vi "Panel Washer Details.vi"(0 "Dryer In":T3 {"Cycle Count" format="%05d"}, 1 "FileName":path caption="Sample Datafilename") -> (4 "Dryer Details Out":T1, 6 "New Filenames":bool)   [LabVIEW 2009]
uses:
  Washer.ctl
  Dryer Wilt/Dryer Details.ctl
  Dryer Wilt/Globals Wilt.vi
panel:
  in  "Return":bool
  out "Array":string[][](array[string])
  out "all rows":string[][](array[string])
  in  "Read Sample Record(t, CC, Tc, ASCII, Status )":string[][](array[string])
  out "L1":dbl[](array[numeric])
  out "Time":dbl[](array[numeric])
  out "Cycle Count":dbl[](array[numeric])
  out "L2":dbl[](array[numeric])
  out "Trmb":dbl[](array[numeric])
  out "Voltage":dbl[](array[numeric])
  in  "Tab Control":T2(tab)
  out "Dryer Details":T1
  out "Display Cycle Count":i32
  out "Station Number":string
  out "Status Color":u32(colorbox)
  out "Bad Com Count":i32
  out "Com Port":u8
  out "Boolean":bool
  out "Sample Plot":cluster{dbl[], dbl[]}[](graph)
  out "Current Cycle Count":dbl
  out "I(L1),I(L2),Trmb,V.V2":dbl[][](array[numeric])
  out "Cycle Count 2":dbl[](array[numeric])
  out "Completion time":dbl[](array[numeric])
  out "L1max":dbl[](array[numeric])
  out "L2max":dbl[](array[numeric])
  out "History Plot":cluster{dbl[], dbl[]}[](graph)
  out "Tmax":dbl[](array[numeric])
  out "Serial Com Array":cluster{dbl, string}[](array[cluster]) {"?" format="%<%H:%M:%S>t"}
  out "Voltage 2":dbl[](array[numeric])
  in  "Update":bool
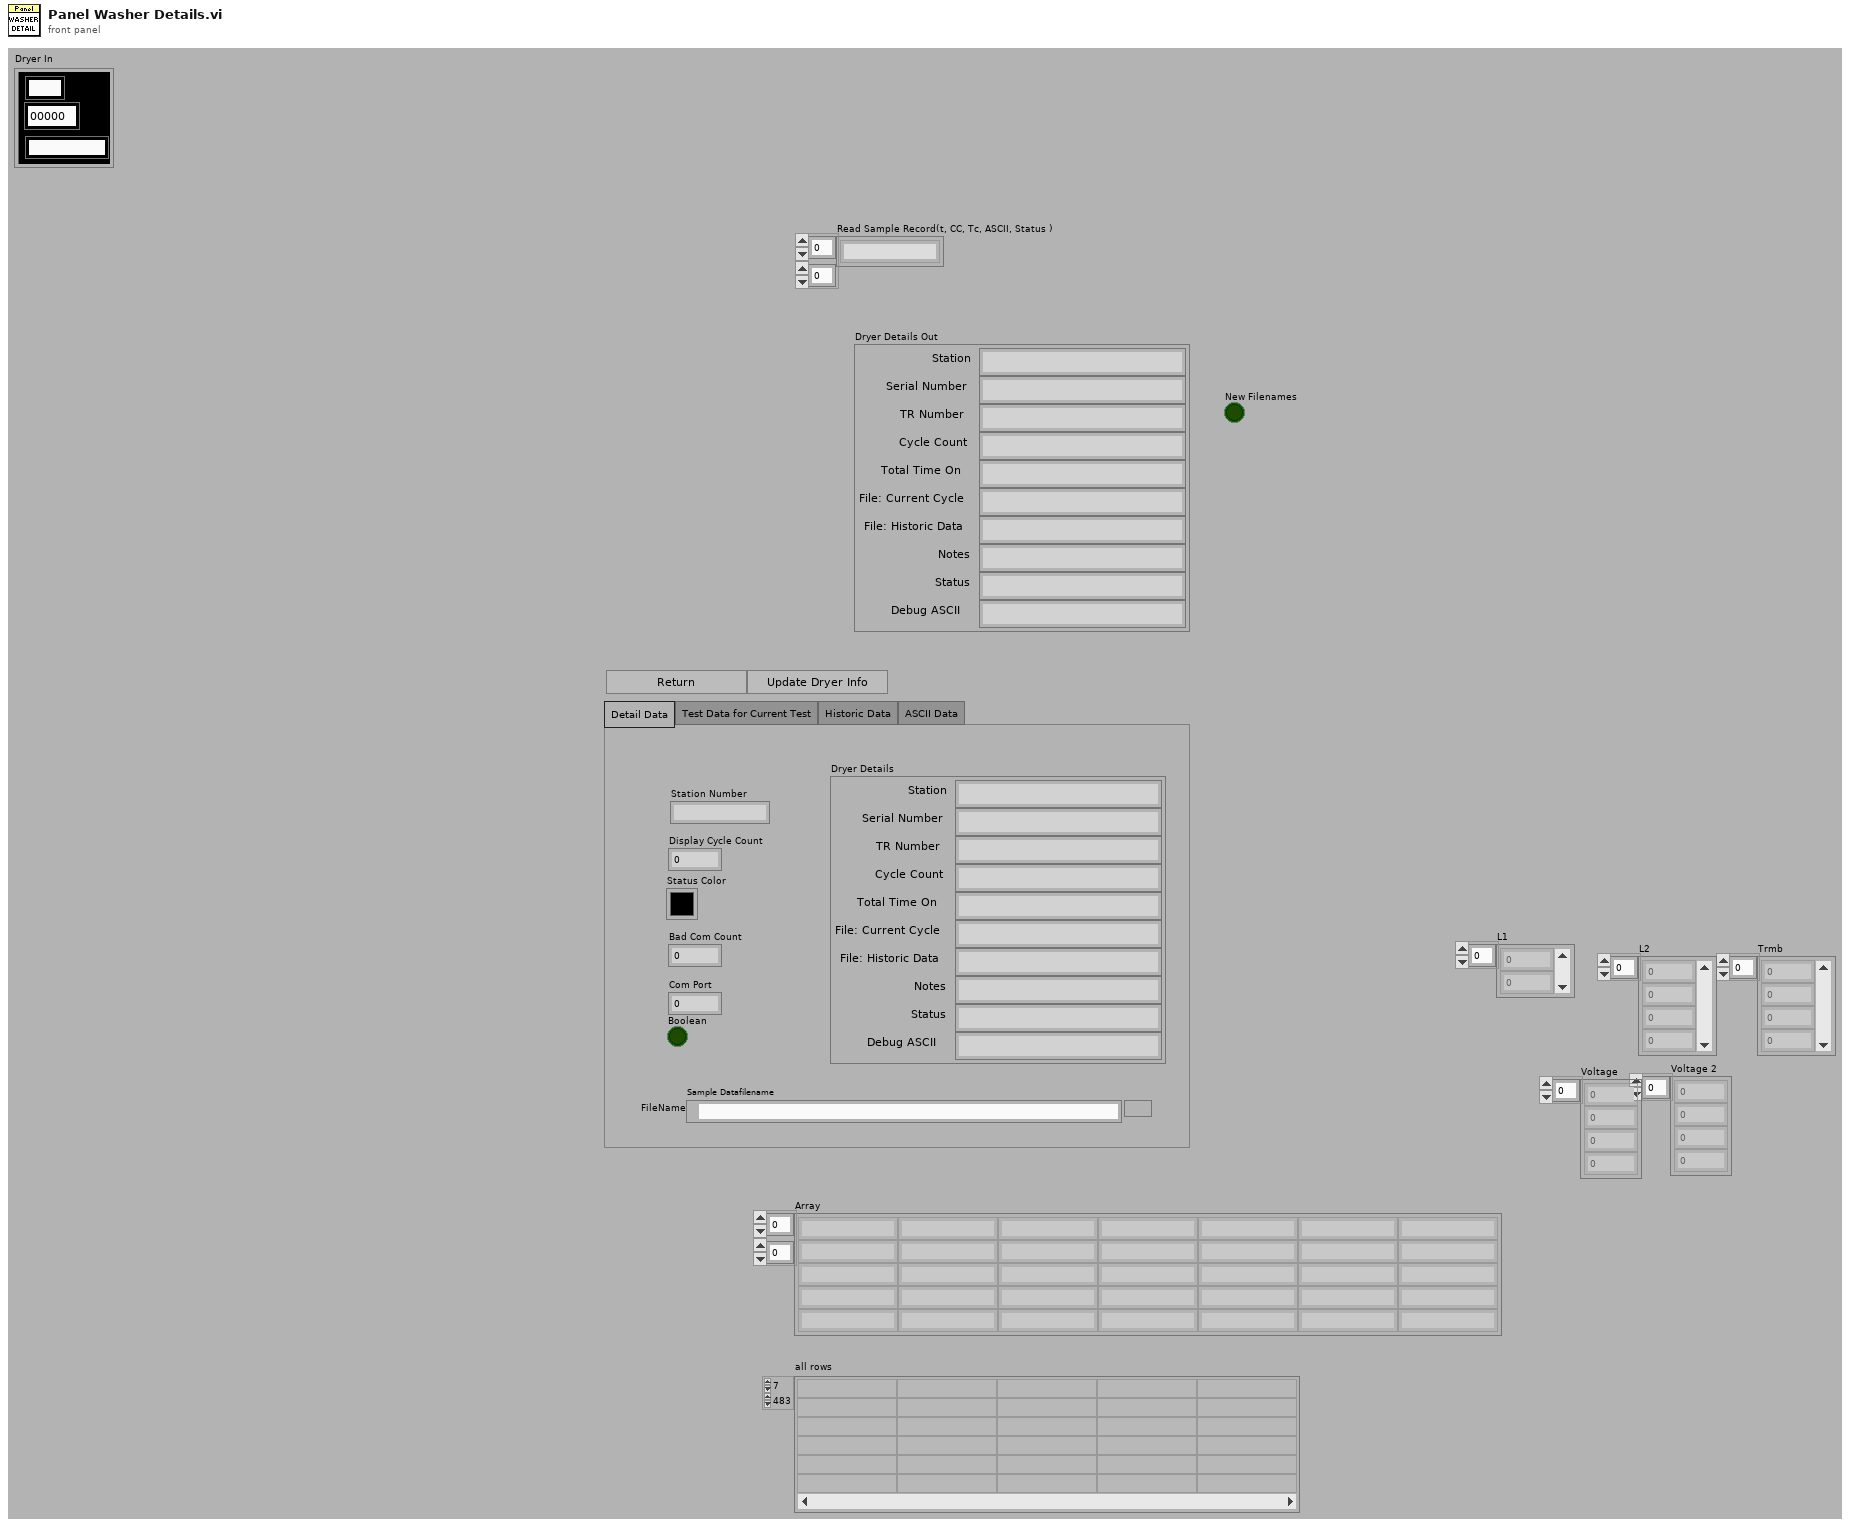
[diagram p1: front panel]
types:
  T1 = typedef "Dryer Details.ctl" = cluster{"Station":string, "Cycle Count":string, "Status":string, "Debug ASCII":string, "Notes":string, "File: Current Cycle":string, "Serial Number":string, "Total Time On":string, "TR Number":string, "File: Historic Data":string}
  T2 = enum32{"Detail Data", "Test Data for Current Test", "Historic Data", "ASCII Data"}
  T3 = typedef "Washer.ctl" = cluster{"Serial Number":string, "Cycle Count":i32, "Station Number":string, "Dryer Details":T1, "Sample Record(t, CC, ASCII, Status ) ":string[], "Hist Record(Cycle Count, t-comp) ":string[][], "Status Color":u32, "Com Port":u8, "Bad Com Count":i32, "Boolean":bool}
  T4 = enum16{"Read 2D Array", "Write 2D Array", "Write/Append 1D Array"}
  T5 = cluster{"FileName":path, "New File Info":bool, "Dryer In":T3, "Read Sample Record(t, CC, Tc, ASCII, Status )":string[][]}
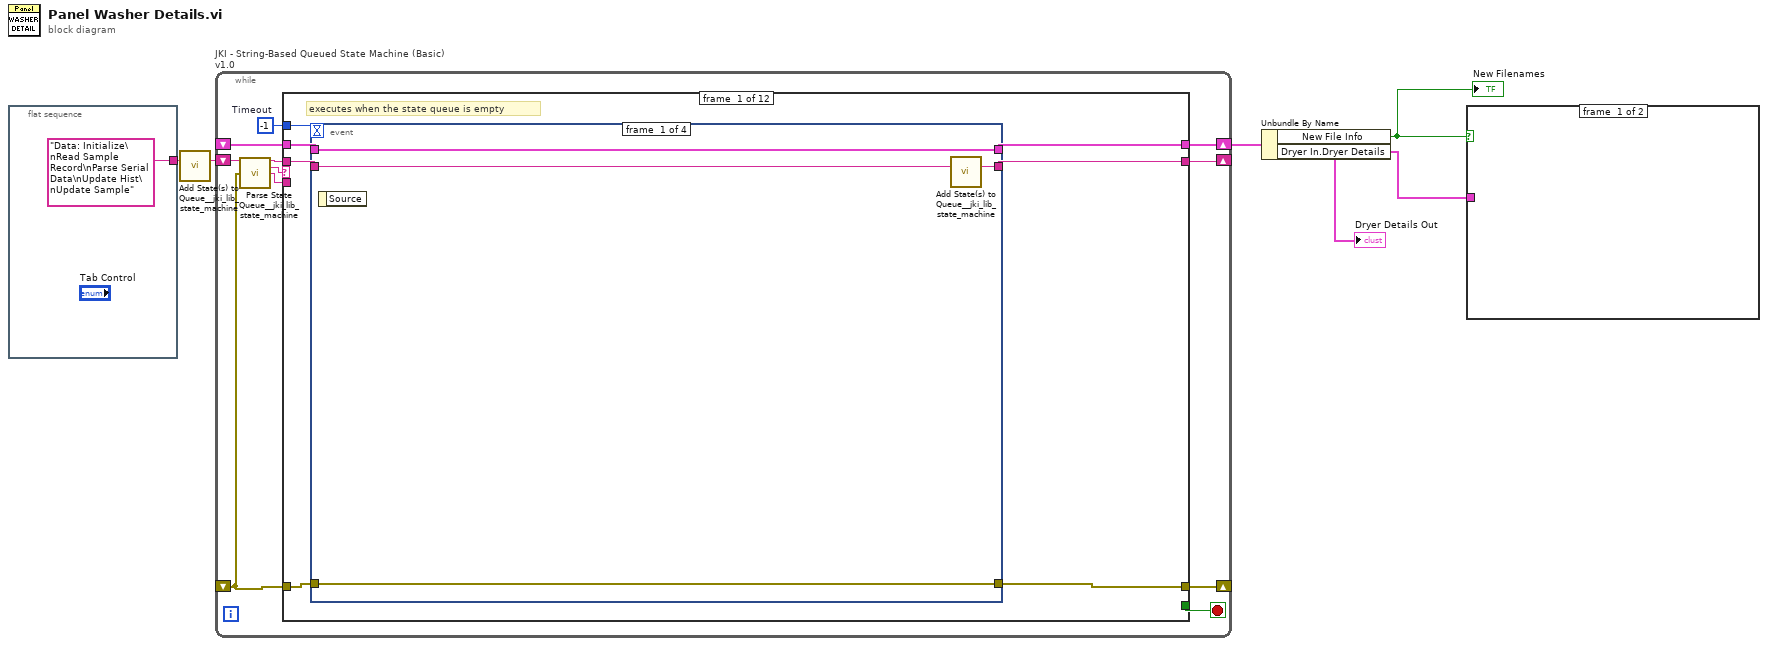
[diagram p0: block diagram]
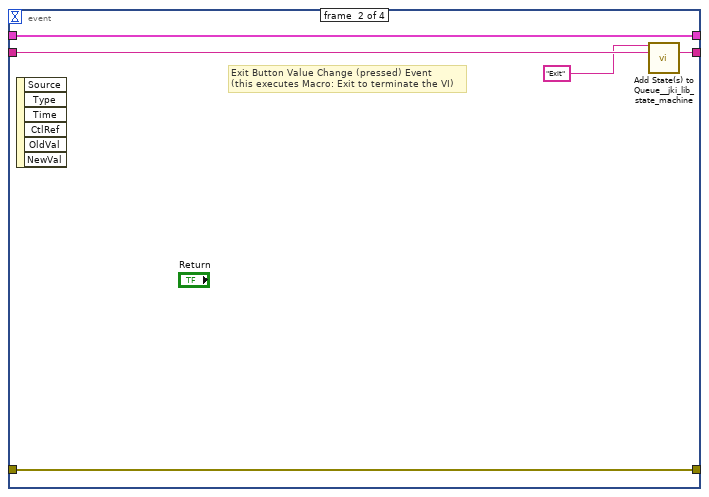
[diagram p2: hidden frame]
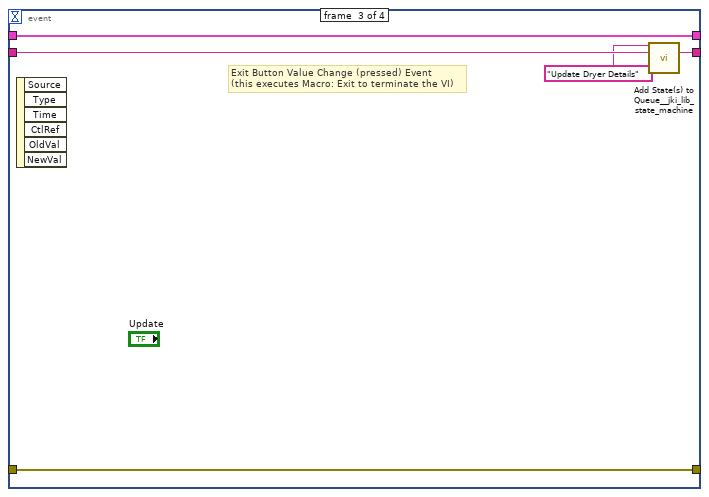
[diagram p3: hidden frame]
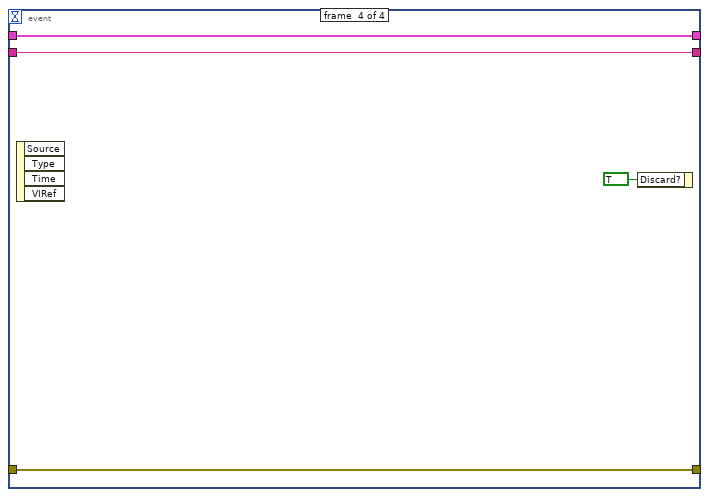
[diagram p4: hidden frame]
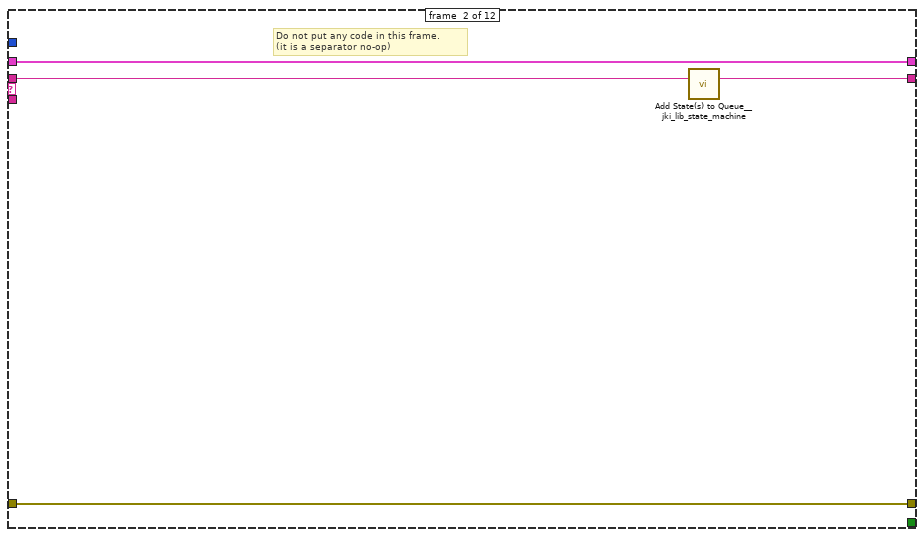
[diagram p5: hidden frame]
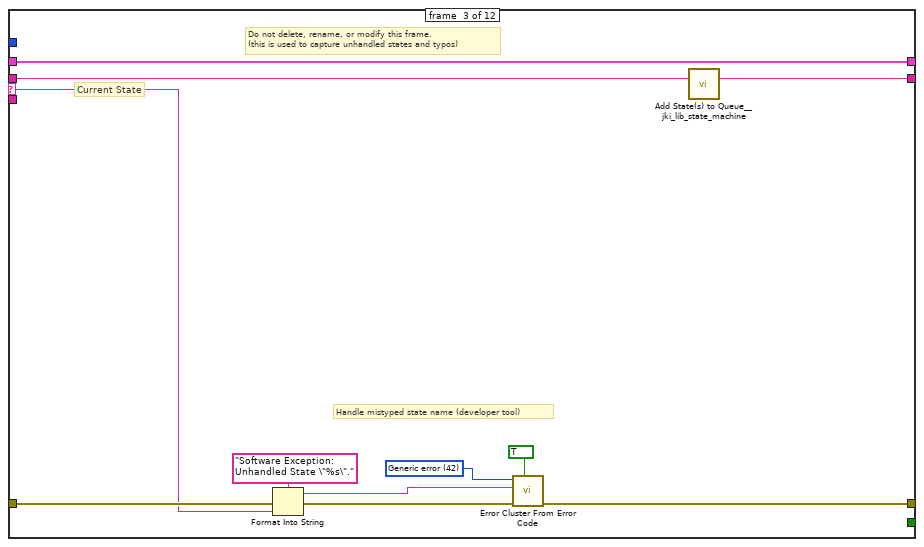
[diagram p6: hidden frame]
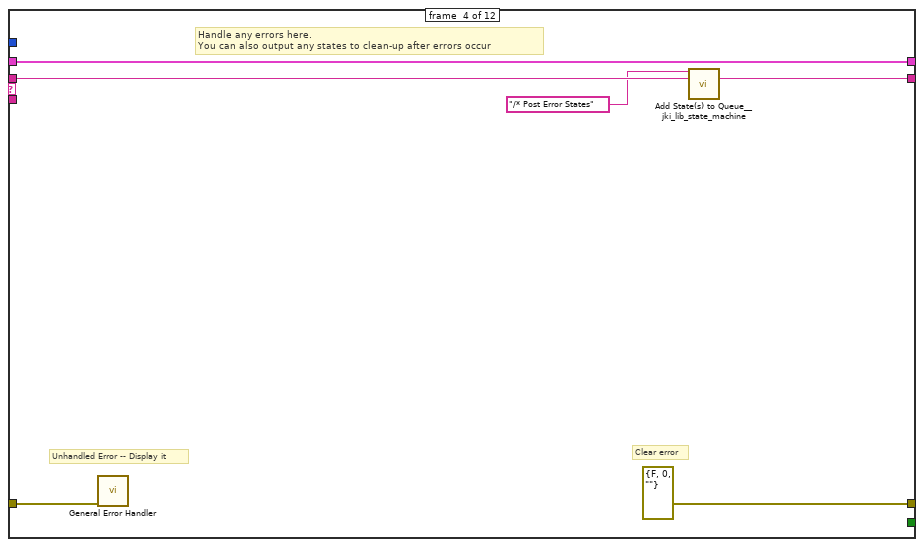
[diagram p7: hidden frame]
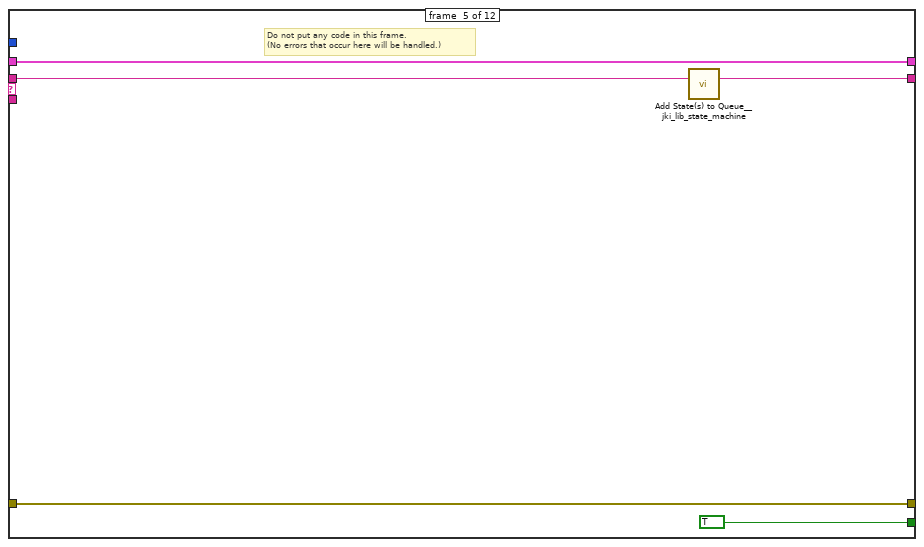
[diagram p8: hidden frame]
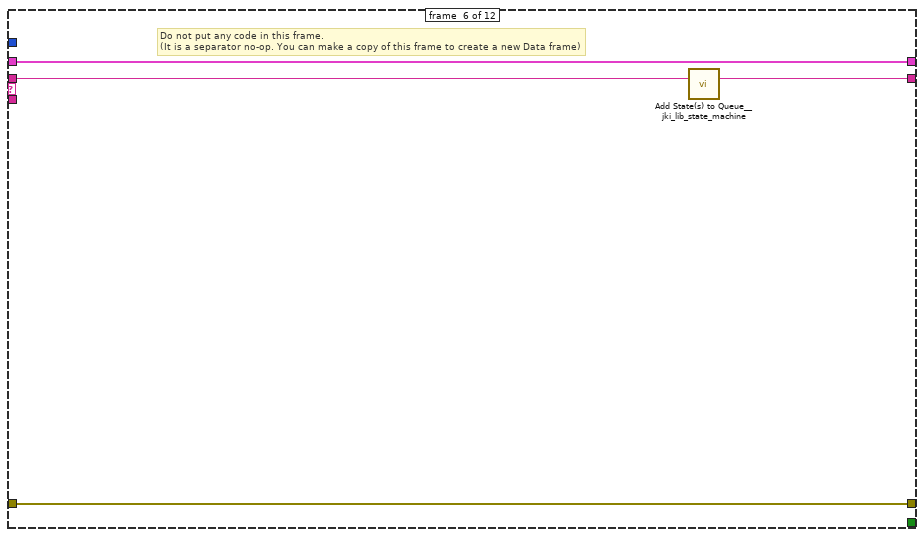
[diagram p9: hidden frame]
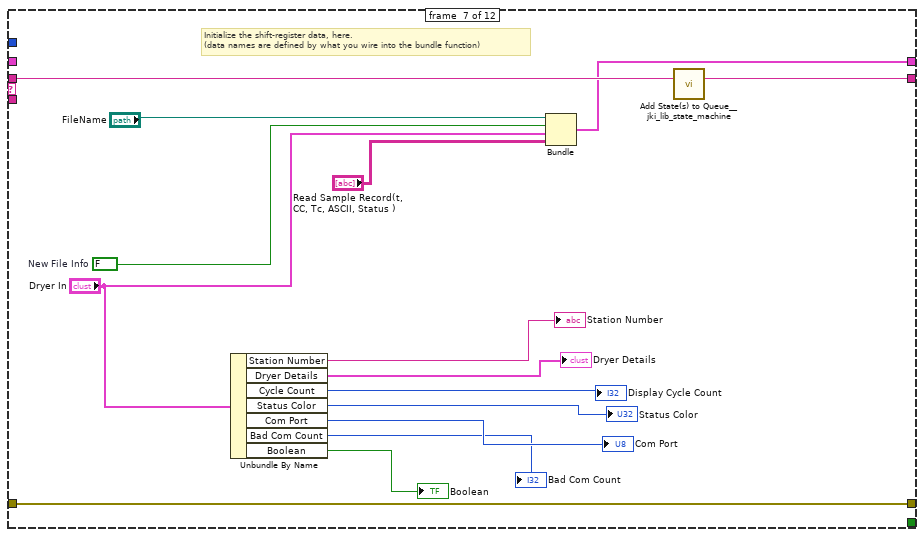
[diagram p10: hidden frame]
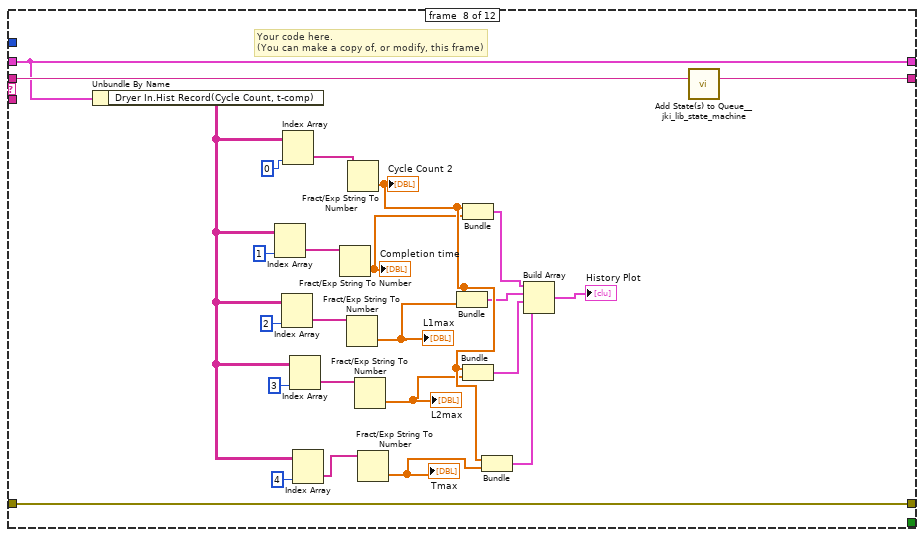
[diagram p11: hidden frame]
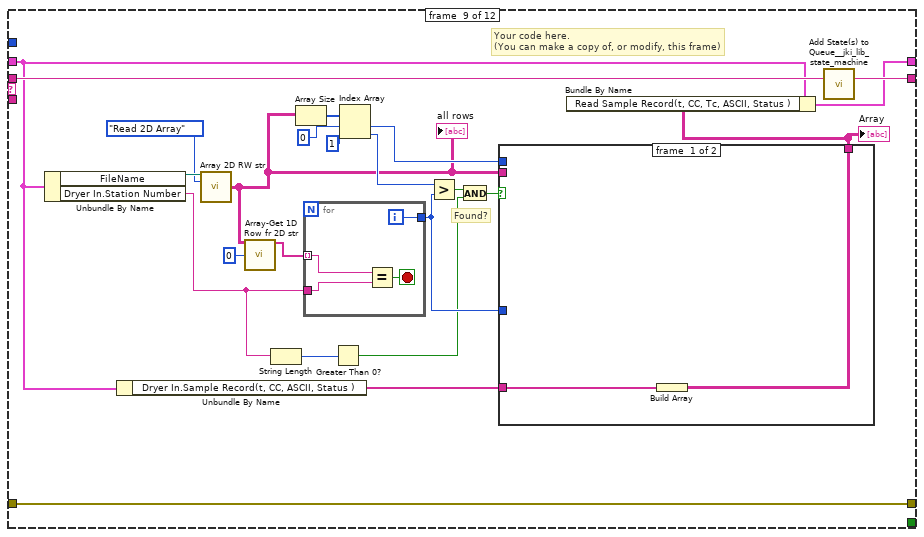
[diagram p12: hidden frame]
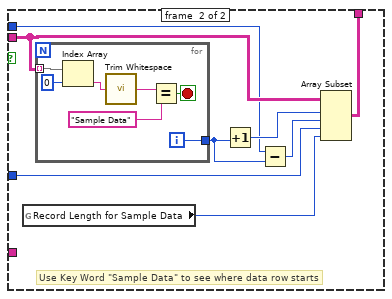
[diagram p13: hidden frame]
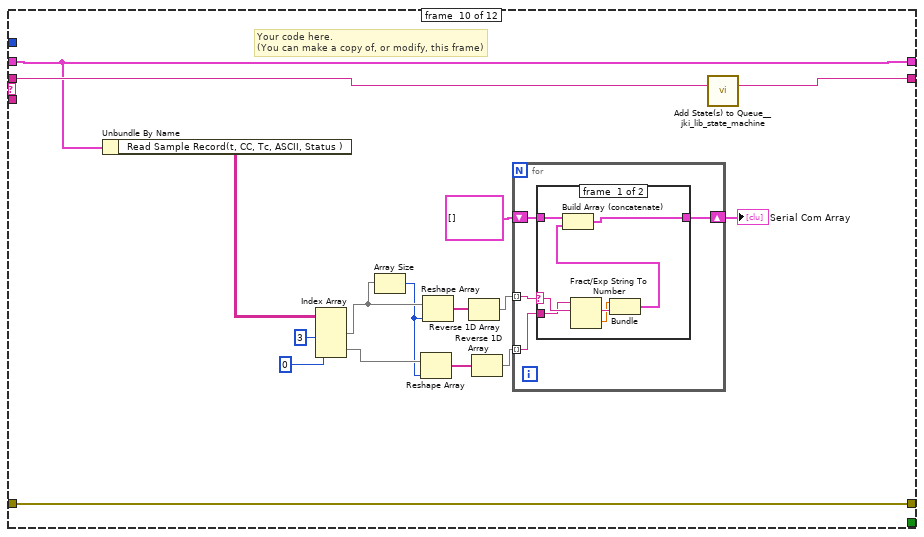
[diagram p14: hidden frame]
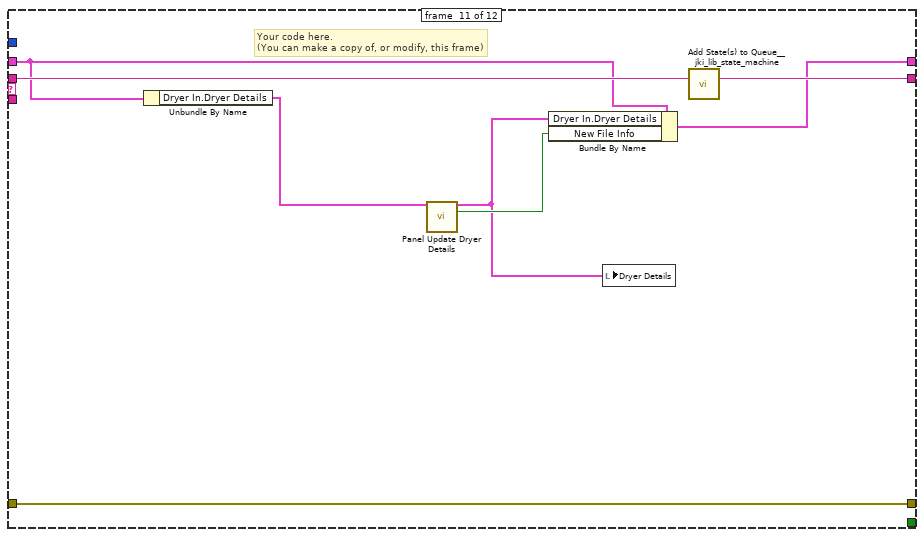
[diagram p16: hidden frame]
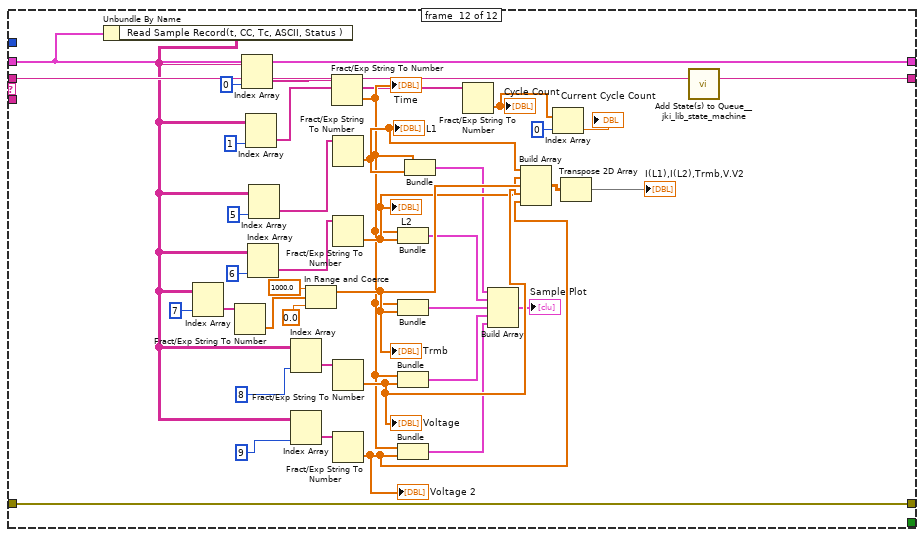
[diagram p17: hidden frame]
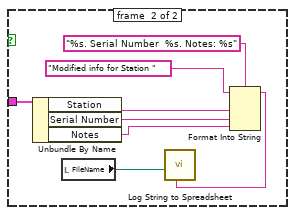
[diagram p18: hidden frame]
diagram:
  n1 = flat-sequence {
    tunnel: ["Data: Initialize\nRead Sample Record\nParse Serial Data\nUpdate Hist\nUpdate Sample"] -> w4
    frame #0 {
    }
  }
  n2 = call <vilib>:"Add State(s) to Queue__jki_lib_state_machine.vi"("State(s) in (\"\")"=w4) -> ("States Out"=w5:string)  [unwired: 14 in]
  n3 = while "JKI - String-Based Queued State Machine (Basic) v1.0" {
    shift-right: [w10] -> w3
    shift-left: _ -> [w9]
    shift-right: [w13] -> _
    shift-left: _ -> [w7]
    shift-right: [w12] -> _
    shift-left: w5 -> [w14]
    stop <- w11 stop-if-true
    w8 = -1  # Timeout
    n4 = call <vilib>:"Parse State Queue__jki_lib_state_machine.vi"("State Queue"=w14, "Error In (no error)"=w7) -> ("Remaining States"=w16:string, "Current State"=w17:string, "Arguments"=w15:string)  [unwired: 11 in]
    n5 = case shown="\"Read Sample Record\"" w17 {
      selector: w17 -> [_ _ w47 _ _ _ _ _ _ _ _ _]
      tunnel: w16 -> [w24 w46 w51 w63 w68 w72 w87 w112 w135 w172 w191 w230]
      tunnel: w15 -> [_ _ _ _ _ _ _ _ _ _ _ _]
      tunnel: w9 -> [w22 w43 w49 w60 w66 w69 _ w89 w129 w169 w187 w193]
      tunnel: [w21 w44 w53 errorcluster {"status"=FALSE, "code"=0, "source"=""} ("error out") w65 w70 w84 w110 w133 w170 w189 w228] -> w13
      tunnel: w7 -> [w20 w44 w52 w59 w65 w70 w84 w110 w133 w170 w189 w228]
      tunnel: [w23 w45 w50 w62 w67 w71 w86 w111 w134 w171 w190 w229] -> w12
      tunnel: [_ _ _ _ TRUE _ _ _ _ _ _ _] -> w11
      tunnel: [w19 w43 w49 w60 w66 w69 w85 w89 w128 w169 w186 w193] -> w10
      tunnel: w8 -> [w18 _ _ _ _ _ _ _ _ _ _ _]
      frame #0 {
        # "executes when the state queue is empty"
        n6 = event shown="[3] Panel Close?" {
          selector: _ -> [_ _ _ _]
          dyn-events: _ -> [_ _ _ _]
          timeout: w18 -> [_ _ _ _]
          tunnel: w24 -> [w28 w33 w38 w41]
          tunnel: [w27 w32 w37 w41] -> w23
          tunnel: w22 -> [w25 w30 w35 w42]
          tunnel: [w26 w31 w36 w39] -> w21
          tunnel: w20 -> [w26 w31 w36 w39]
          tunnel: [w25 w30 w35 w42] -> w19
          event #0 {
            n7 = event-data() -> ()  [unwired: 1 in, 1 out]
            n8 = call <vilib>:"Add State(s) to Queue__jki_lib_state_machine.vi"("State(s) in (\"\")"=w28) -> ("States Out"=w27:string)  [unwired: 14 in]
          }
          event #1 {
            # "Exit Button Value Change (pressed) Event\n(this executes Macro: Exit to terminate the VI)"
            n9 = event-data() -> ()  [unwired: 1 in, 6 out]
            n10 = call <vilib>:"Add State(s) to Queue__jki_lib_state_machine.vi"("State(s) in Front (\"\")"="Exit", "State(s) in (\"\")"=w33) -> ("States Out"=w32:string)  [unwired: 13 in]
          }
          event #2 {
            # "Exit Button Value Change (pressed) Event\n(this executes Macro: Exit to terminate the VI)"
            n11 = event-data() -> ()  [unwired: 1 in, 6 out]
            n12 = call <vilib>:"Add State(s) to Queue__jki_lib_state_machine.vi"("State(s) in Front (\"\")"="Update Dryer Details", "State(s) in (\"\")"=w38) -> ("States Out"=w37:string)  [unwired: 13 in]
          }
          event #3 {
            n13 = event-data() -> ()  [unwired: 1 in, 4 out]
            n14 = event-data("Discard?"=TRUE) -> ()  [unwired: 1 in, 1 out]
          }
        }
      }
      frame #1 {
        # "Do not put any code in this frame.\n(it is a separator no-op)"
        n15 = call <vilib>:"Add State(s) to Queue__jki_lib_state_machine.vi"("State(s) in (\"\")"=w46) -> ("States Out"=w45:string)  [unwired: 14 in]
      }
      frame #2 {
        w56 = 42 items=["No error", "Argument error", "Memory is full", "Out of zone", "End of file", "File already open", "Generic file I/O error", "File not found", "File permission error", "Disk is full", "Duplicate path", "Too many files open", "System feature not enabled", "Resource file not found", "Cannot add resource", "Resource not found", "Image not found", "Image memory error", "Pen does not exist", "Config type invalid", "Config token not found", "Config parse error", "Config memory error", "Bad external code format", "Bad external code offset", "External code not present", "Null window", "Destroy window error", "Null menu", "Print aborted", "Bad print record", "Print driver error", "Windows error during printing", "Memory error during printing", "Print dialog error", "Generic print error", "Invalid device refnum", "Device not found", "Device parameter error", "Device unit error", "Cannot open device", "Device call aborted", "Generic error", "Cancelled by user", "Object ID too low", "Object ID too high", "Object not in heap", "Unknown heap", "Unknown object (invalid DefProc)", "Unknown object (DefProc not in table)", "Message out of range", "Invalid (null) method", "Unknown message", "Manager call not supported", "Bad address", "Network operation in progress", "Network operation timed out", "Connection is busy", "Network attribute not supported", "Network error", "Address in use", "System out of memory", "Connection aborted", "Connection refused", "Not connected", "Already connected", "Connection closed", "Initialization error (interapplication manager)", "Bad occurrence", "Wait on unbound occurrence handler", "Occurrence queue overflow", "Datalog type conflict", "Unused", "Unrecognized type (interapplication manager)", "Memory corrupt", "Failed to make temporary DLL", "Old CIN version", "Drag socket not found", "Failed to load drop-object", "Failed to register OLE object", "Failed to release OLE object", "Format specifier type mismatch", "Unknown format specifier", "Too few format specifiers", "Too many format specifiers", "Scan failed", "Newer CIN version", "Error converting to variant", "Runtime menu error", "Password tampered", "Variant attribute not found", "Incompatible variant data type", "Event data is not available", "Event Store is not present", "Occurrence is not found", "Event Queue is not created", "Event info is not available", "Refnum passed is NULL", "Error retrieving Class GUID", "Error retrieving CoClass GUID", "Error retrieving TypeLib GUID.", "Bad built application magic bytes.", "Specific driver is different from the specific driver associated with the Logical Name.", "There is no session opened to the class driver.", "Max Error", "MAX - Error with config objects", "MAX - Error loading configuration", "MAX - Group not supported"]
        # "Current State"
        # "Do not delete, rename, or modify this frame.\n(this is used to capture unhandled states and typos)"
        # "Handle mistyped state name (developer tool)"
        n16 = Format Into String(format string="Software Exception: Unhandled State \"%s\"." ("message"), error in=w52, w47) -> (resulting string=w55:string, error out=w54:errorcluster)  [unwired: 1 in]
        n17 = call <vilib>:"Error Cluster From Error Code.vi"("show call chain? (False)"=TRUE, "error in (no error)"=w54, "error message (\"\")"=w55, "error code (0)"=w56) -> ("error out"=w53:errorcluster)  [unwired: 5 in]
        n18 = call <vilib>:"Add State(s) to Queue__jki_lib_state_machine.vi"("State(s) in (\"\")"=w51) -> ("States Out"=w50:string)  [unwired: 14 in]
      }
      frame #3 {
        # "Unhandled Error -- Display it"
        # "Handle any errors here.\nYou can also output any states to clean-up after errors occur"
        # "Clear error"
        n19 = call <vilib>:"General Error Handler.vi"("error in (no error)"=w59) -> ()  [unwired: 10 in, 5 out]
        n20 = call <vilib>:"Add State(s) to Queue__jki_lib_state_machine.vi"("State(s) in Front (\"\")"="/* Post Error States", "State(s) in (\"\")"=w63) -> ("States Out"=w62:string)  [unwired: 13 in]
      }
      frame #4 {
        # "Do not put any code in this frame.\n(No errors that occur here will be handled.)"
        n21 = call <vilib>:"Add State(s) to Queue__jki_lib_state_machine.vi"("State(s) in (\"\")"=w68) -> ("States Out"=w67:string)  [unwired: 14 in]
      }
      frame #5 {
        # "Do not put any code in this frame.\n(It is a separator no-op. You can make a copy of this frame to create a new Data frame)"
        n22 = call <vilib>:"Add State(s) to Queue__jki_lib_state_machine.vi"("State(s) in (\"\")"=w72) -> ("States Out"=w71:string)  [unwired: 14 in]
      }
      frame #6 {
        w83 = FALSE  # New File Info
        # "Initialize the shift-register data, here.\n(data names are defined by what you wire into the bundle function)"
        n23 = Unbundle By Name("Dryer In") -> ("Station Number"=→"Station Number":string, "Dryer Details"=→"Dryer Details":T1, "Cycle Count"=→"Display Cycle Count":i32, "Status Color"=→"Status Color":u32, "Com Port"=→"Com Port":u8, "Bad Com Count"=→"Bad Com Count":i32, "Boolean"=→"Boolean":bool)
        n24 = Bundle("FileName"="FileName", "New File Info"=w83, "Dryer In"="Dryer In", "Read Sample Record(t, CC, Tc, ASCII, Status )"="Read Sample Record(t, CC, Tc, ASCII, Status )") -> (w85:T5)  [unwired: 1 in]
        n25 = call <vilib>:"Add State(s) to Queue__jki_lib_state_machine.vi"("State(s) in (\"\")"=w87) -> ("States Out"=w86:string)  [unwired: 14 in]
      }
      frame #7 {
        # "Your code here.\n(You can make a copy of, or modify, this frame)"
        n26 = Unbundle By Name(w89) -> ("Dryer In.Hist Record(Cycle Count, t-comp)"=w88:string[][])
        n27 = Index Array(array=w88, index (col)=1 ("disabled index (col)")) -> (element=w92:string[])  [unwired: 1 in]
        n28 = Index Array(array=w88, index (col)=2 ("disabled index (col)")) -> (element=w93:string[])  [unwired: 1 in]
        n29 = Index Array(array=w88, index (col)=0 ("disabled index (col)")) -> (element=w90:string[])  [unwired: 1 in]
        n30 = Index Array(array=w88, index (col)=3 ("disabled index (col)")) -> (element=w97:string[])  [unwired: 1 in]
        n31 = Index Array(array=w88, index (col)=4 ("disabled index (col)")) -> (element=w106:string[])  [unwired: 1 in]
        n32 = Fract/Exp String To Number(string=w92) -> (number=w98:dbl[])  [unwired: 3 in, 1 out]
        "Completion time" <- w98
        n33 = Fract/Exp String To Number(string=w93) -> (number=w99:dbl[])  [unwired: 3 in, 1 out]
        "L1max" <- w99
        n34 = Fract/Exp String To Number(string=w90) -> (number=w108:dbl[])  [unwired: 3 in, 1 out]
        "Cycle Count 2" <- w108
        n35 = Fract/Exp String To Number(string=w97) -> (number=w100:dbl[])  [unwired: 3 in, 1 out]
        "L2max" <- w100
        n36 = Fract/Exp String To Number(string=w106) -> (number=w107:dbl[])  [unwired: 3 in, 1 out]
        "Tmax" <- w107
        n37 = Bundle(w108, w99) -> (w103:cluster{dbl[], dbl[]})  [unwired: 1 out]
        n38 = Bundle(w108, w98) -> (w102:cluster{dbl[], dbl[]})  [unwired: 1 out]
        n39 = Bundle(w108, w100) -> (w104:cluster{dbl[], dbl[]})  [unwired: 1 out]
        n40 = Bundle(w108, w107) -> (w109:cluster{dbl[], dbl[]})  [unwired: 1 out]
        n41 = Build Array(w102, w103, w104, w109) -> (→"History Plot":cluster{dbl[], dbl[]}[])
        n42 = call <vilib>:"Add State(s) to Queue__jki_lib_state_machine.vi"("State(s) in (\"\")"=w112) -> ("States Out"=w111:string)  [unwired: 14 in]
      }
      frame #8 {
        # "Found?"
        # "Your code here.\n(You can make a copy of, or modify, this frame)"
        n43 = Unbundle By Name(w129) -> ("FileName"=w116:path, "Dryer In.Station Number"=w124:string)
        n44 = Unbundle By Name(w129) -> ("Dryer In.Sample Record(t, CC, ASCII, Status )"=w122:string[])
        n45 = call "Array 2D RW str.vi"("file path (dialog if empty)"=w116, "Write/Read"=T4."Read 2D Array") -> ("Read all rows"=w115:string[][])  [unwired: 13 in]
        "all rows" <- w115
        n46 = call "Array-Get 1D Row fr 2D str.vi"("all rows"=w115, "row index"=0) -> ("row"=w119:string[])  [unwired: 13 in]
        n47 = String Length(string=w124) -> (length=w113:i32)
        n48 = Array Size(array=w115) -> (size(s)=w132:i32[])
        n49 = for {
          tunnel: w119 -> [w154] mode=indexing
          tunnel: w124 -> [w153]
          tunnel: [w155] -> w130
          i -> [w155]
          stop <- w156 stop-if-true
          n50 = Equal?(x=w154, y=w153) -> (x = y?=w156:bool)
        }
        n51 = Greater Than 0?(x=w113) -> (x > 0?=w123:bool)
        n52 = Index Array(array=w132, index #1=0 ("index"), index #2=1 ("index")) -> (element #1=w117:i32, element #2=w120:i32)
        n53 = Greater?(x=w120, y=w130) -> (0:w126:bool)
        n54 = And(x=w126, y=w123) -> (x .and. y?=w125:bool)
        n55 = case shown="True" w125 {
          tunnel: w115 -> [_ w144]
          tunnel: w130 -> [_ w143]
          tunnel: [w136 w142] -> w127
          tunnel: w122 -> [w137 _]
          tunnel: w117 -> [_ w139]
          frame #0 {
            n56 = Build Array(w137) -> (w136:string[][])
          }
          frame #1 {
            # "Use Key Word \"Sample Data\" to see where data row starts"
            n57 = global read "Globals Wilt.vi" "Record Length for Sample Data"() -> (w141:i32)
            n58 = for {
              tunnel: w144 -> [w152] mode=indexing
              tunnel: [w149] -> w138
              i -> [w149]
              stop <- w148 stop-if-true
              n59 = Index Array(array=w152, index=0) -> (element=w147:string)
              n60 = call <vilib>:"Trim Whitespace.vi"("string"=w147) -> ("trimmed string"=w146:string)  [unwired: 1 in]
              n61 = Equal?(x=w146, y="Sample Data") -> (x = y?=w148:bool)
            }
            n62 = Increment(x=w138) -> (x+1=w145:i32)
            n63 = Subtract(x=w139, y=w138) -> (x-y=w140:i32)
            n64 = Array Subset(array=w144, index (row)=w145, length (row)=w140, index (col)=w143, length (col)=w141) -> (w142:string[][])
          }
        }
        "Array" <- w127
        n65 = Bundle By Name(cluster=w129, "Read Sample Record(t, CC, Tc, ASCII, Status )"=w127) -> (w128:T5)
        n66 = call <vilib>:"Add State(s) to Queue__jki_lib_state_machine.vi"("State(s) in (\"\")"=w135) -> ("States Out"=w134:string)  [unwired: 14 in]
      }
      frame #9 {
        # "Your code here.\n(You can make a copy of, or modify, this frame)"
        n67 = Unbundle By Name(w169) -> ("Read Sample Record(t, CC, Tc, ASCII, Status )"=w159:string[][])
        n68 = Index Array(array=w159, index (col) #1=3 ("disabled index (col)"), index (col) #2=0 ("index (col)")) -> (element #1=w158:string[], element #2=w165:string[])  [unwired: 2 in]
        n69 = Array Size(array=w158) -> (size(s)=w157:i32)
        n70 = Reshape Array(w165, w157) -> (w164:string[])
        n71 = Reshape Array(w158, w157) -> (w167:string[])
        n72 = Reverse 1D Array(array=w167) -> (reversed array=w163:string[])
        n73 = Reverse 1D Array(array=w164) -> (reversed array=w162:string[])
        n74 = for {
          tunnel: w163 -> [w176] mode=indexing
          tunnel: w162 -> [w175] mode=indexing
          shift-right: [w174] -> w161
          shift-left: cluster{dbl, string}[] [] -> [w173]
          n75 = case shown="\"Data\", Default" w176 {
            selector: w176 -> [w182 _]
            tunnel: w175 -> [w181 _]
            tunnel: [w179 w183] -> w174
            tunnel: w173 -> [w178 w183]
            frame #0 {
              n76 = Fract/Exp String To Number(string=w181) -> (number=w177:dbl)  [unwired: 3 in, 1 out]
              n77 = Bundle(w177, w182) -> (w180:cluster{dbl, string})  [unwired: 1 in]
              n78 = Build Array (concatenate)(w178, w180) -> (w179:cluster{dbl, string}[])
            }
            frame #1 {
            }
          }
        }
        "Serial Com Array" <- w161
        n79 = call <vilib>:"Add State(s) to Queue__jki_lib_state_machine.vi"("State(s) in (\"\")"=w172) -> ("States Out"=w171:string)  [unwired: 14 in]
      }
      frame #10 {
        # "Your code here.\n(You can make a copy of, or modify, this frame)"
        n80 = Unbundle By Name(w187) -> ("Dryer In.Dryer Details"=w188:T1)
        n81 = call "Panel Update Dryer Details.vi"("Dryer Details In"=w188) -> ("Dryer Details Out"=w184:T1, "New Filenames"=w185:bool)  [unwired: 13 in]
        n82 = Bundle By Name(cluster=w187, "Dryer In.Dryer Details"=w184, "New File Info"=w185) -> (w186:T5)
        n83 = local write "Dryer Details"(w184) -> ()
        n84 = call <vilib>:"Add State(s) to Queue__jki_lib_state_machine.vi"("State(s) in (\"\")"=w191) -> ("States Out"=w190:string)  [unwired: 14 in]
      }
      frame #11 {
        n85 = Unbundle By Name(w193) -> ("Read Sample Record(t, CC, Tc, ASCII, Status )"=w192:string[][])
        n86 = Index Array(array=w192, index (col)=7 ("disabled index (col)")) -> (element=w202:string[])  [unwired: 1 in]
        n87 = Fract/Exp String To Number(string=w202) -> (number=w218:dbl[])  [unwired: 3 in, 1 out]
        n88 = Index Array(array=w192, index (col)=0 ("disabled index (col)")) -> (element=w195:string[])  [unwired: 1 in]
        n89 = Index Array(array=w192, index (col)=1 ("disabled index (col)")) -> (element=w196:string[])  [unwired: 1 in]
        n90 = Index Array(array=w192, index (col)=6 ("disabled index (col)")) -> (element=w199:string[])  [unwired: 1 in]
        n91 = Index Array(array=w192, index (col)=5 ("disabled index (col)")) -> (element=w197:string[])  [unwired: 1 in]
        n92 = Index Array(array=w192, index (col)=8 ("disabled index (col)")) -> (element=w204:string[])  [unwired: 1 in]
        n93 = Index Array(array=w192, index (col)=9 ("disabled index (col)")) -> (element=w206:string[])  [unwired: 1 in]
        n94 = In Range and Coerce(upper limit=1000.0 ("String"), x=w218, lower limit=0.0 ("String")) -> (coerced(x)=w223:dbl[])  [unwired: 1 out]
        "Trmb" <- w223
        n95 = Fract/Exp String To Number(string=w195) -> (number=w208:dbl[])  [unwired: 3 in, 1 out]
        "Time" <- w208
        n96 = Fract/Exp String To Number(string=w197) -> (number=w221:dbl[])  [unwired: 3 in, 1 out]
        "L1" <- w221
        n97 = Fract/Exp String To Number(string=w199) -> (number=w222:dbl[])  [unwired: 3 in, 1 out]
        "L2" <- w222
        n98 = Fract/Exp String To Number(string=w204) -> (number=w224:dbl[])  [unwired: 3 in, 1 out]
        "Voltage" <- w224
        n99 = Fract/Exp String To Number(string=w206) -> (number=w225:dbl[])  [unwired: 3 in, 1 out]
        "Voltage 2" <- w225
        n100 = Bundle(w208, w222) -> (w209:cluster{dbl[], dbl[]})  [unwired: 1 out]
        n101 = Bundle(w208, w223) -> (w211:cluster{dbl[], dbl[]})  [unwired: 1 out]
        n102 = Bundle(w208, w224) -> (w212:cluster{dbl[], dbl[]})  [unwired: 1 out]
        n103 = Bundle(w208, w225) -> (w213:cluster{dbl[], dbl[]})  [unwired: 1 out]
        n104 = Bundle(w208, w221) -> (w210:cluster{dbl[], dbl[]})  [unwired: 1 out]
        n105 = Fract/Exp String To Number(string=w196) -> (number=w215:dbl[])  [unwired: 3 in, 1 out]
        "Cycle Count" <- w215
        n106 = Build Array(w210, w209, w211, w212, w213) -> (→"Sample Plot":cluster{dbl[], dbl[]}[])
        n107 = Build Array(w221, w222, w223, w224, w225) -> (w226:dbl[][])
        n108 = Index Array(array=w215, index=0) -> (element=→"Current Cycle Count":dbl)
        n109 = Transpose 2D Array(2D array=w226) -> (transposed array=→"I(L1),I(L2),Trmb,V.V2":dbl[][])
        n110 = call <vilib>:"Add State(s) to Queue__jki_lib_state_machine.vi"("State(s) in (\"\")"=w230) -> ("States Out"=w229:string)  [unwired: 14 in]
      }
    }
  }
  n111 = Unbundle By Name(w3) -> ("New File Info"=w1:bool, "Dryer In.Dryer Details"=w2:T1)
  "Dryer Details Out" <- w2
  "New Filenames" <- w1
  n112 = case shown="True" w1 {
    tunnel: w2 -> [_ w237]
    frame #0 {
    }
    frame #1 {
      n113 = Unbundle By Name(w237) -> ("Station"=w236:string, "Serial Number"=w234:string, "Notes"=w233:string)
      n114 = local read "FileName"() -> (w231:path)
      n115 = Format Into String(format string="%s. Serial Number  %s. Notes: %s", initial string="Modified info for Station ", w236, w234, w233) -> (resulting string=w232:string)  [unwired: 1 in, 1 out]
      n116 = call "Log String to Spreadsheet.vi"("String"=w232, "FileName"=w231) -> ()  [unwired: 9 in, 1 out]
    }
  }
